vi "Xsens DT Parser (SubVI).vi"(5 "DT String In":string, 6 "DataType In":string) -> (0 "Channel Units":string[](array[string]), 1 "Channel DataTypes":string[](array[string]), 2 "Decoded Data Out":string[](array[string]), 3 "Channel Names":string[](array[string]))   [LabVIEW 2019]
doc: "This SubVI uses a state machine type structure to decode the XSens data measurement string based on the provided datatype. It outputs 4 fields that are contain the decoded data and metadata for writing to a TDMS file. \n\nAll data are output as strings. This is necessary to simplify the TDMS write function, since TDMS does not handle mixed data types (float, int, string, bool, etc) easily. \n\nCurrently, does not include decoders for all Xsens datatypes, however decoders can be easily added as need arises. \n\n2020 NREL"
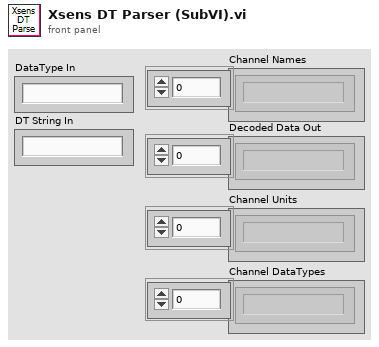
[diagram p1: front panel]
types:
  T1 = cluster{"Valid Time of Week":bool, "Valid Week Number":bool, "Valid UTC":bool}
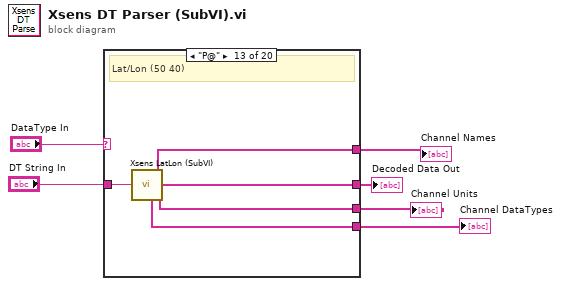
[diagram p0: block diagram]
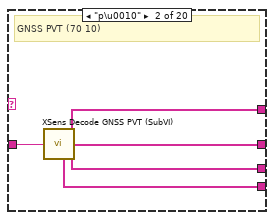
[diagram p3: hidden frame]
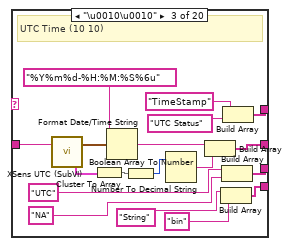
[diagram p4: hidden frame]
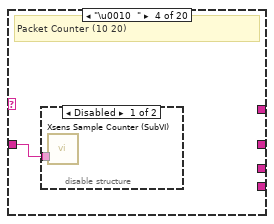
[diagram p5: hidden frame]
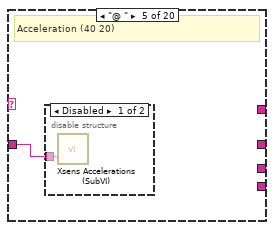
[diagram p7: hidden frame]
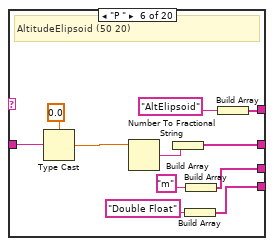
[diagram p9: hidden frame]
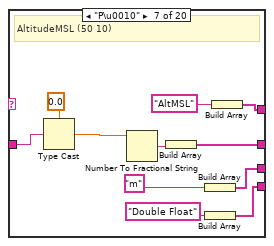
[diagram p10: hidden frame]
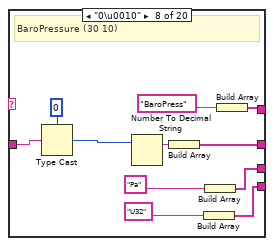
[diagram p11: hidden frame]
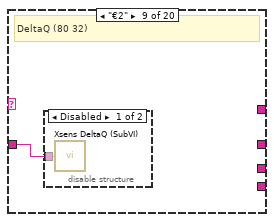
[diagram p12: hidden frame]
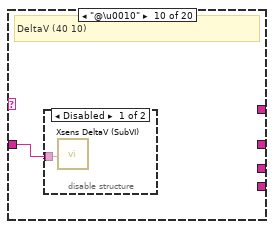
[diagram p14: hidden frame]
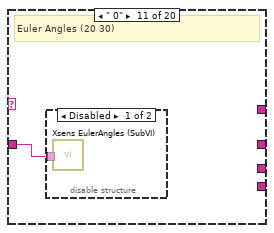
[diagram p16: hidden frame]
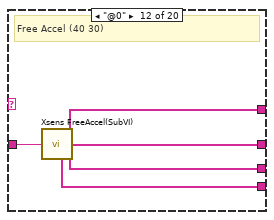
[diagram p18: hidden frame]
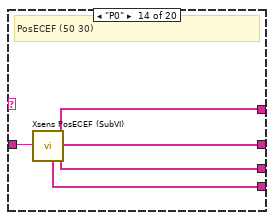
[diagram p19: hidden frame]
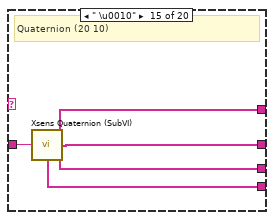
[diagram p20: hidden frame]
diagram:
  n1 = case shown="\"P@\"" "DataType In" {
    tunnel: "DT String In" -> [_ w11 w29 w30 w32 w43 w54 w65 w67 w69 w71 w77 w82 w87 w92 w97 w98 w100 w103 w110]
    tunnel: [_ w10 w26 _ _ w40 w51 w62 _ _ _ w76 w81 w83 w91 w96 _ _ _ w109] -> w3
    tunnel: [_ w9 w19 _ _ w38 w47 w58 _ _ _ w75 w80 w86 w90 w95 _ _ _ w108] -> w4
    tunnel: [_ w7 w15 _ _ w34 w45 w56 _ _ _ w73 w79 w84 w88 w93 _ _ _ w106] -> w1
    tunnel: [_ w8 w17 _ _ w35 w46 w57 _ _ _ w74 w78 w85 w89 w94 _ _ _ w107] -> w2
    frame "False", Default {
    }
    frame "p\u0010" {
      # "GNSS PVT (70 10)"
      n2 = call "XSens Decode GNSS PVT (SubVI).vi"("DATA In (Hex )"=w11) -> ("Channel Units"=w8:string[], "Channel DataTypes"=w7:string[], "GPS PVT out"=w10:string[], "Channel Names"=w9:string[])  [unwired: 1 out]
    }
    frame "\u0010\u0010" {
      # "UTC Time (10 10)"
      n3 = call "XSens UTC (SubVI).vi"("DATA In (Hex)"=w29) -> ("UTC Time"=w28:timestamp, "UTC Time Status"=w24:T1)
      n4 = Cluster To Array(cluster=w24) -> (array=w23:bool[])
      n5 = Format Date/Time String(time format string (%c)="%Y%m%d-%H:%M:%S%6u", seconds (now)=w28) -> (date/time string=w27:string)  [unwired: 1 in]
      n6 = Boolean Array To Number(Boolean array=w23) -> (number=w21:u32)
      n7 = Number To Decimal String(number=w21) -> (decimal integer string=w22:string)  [unwired: 1 in]
      n8 = Build Array(w27, w22) -> (w26:string[])
      n9 = Build Array("String", "bin") -> (w15:string[])
      n10 = Build Array("UTC", "NA") -> (w17:string[])
      n11 = Build Array("TimeStamp", "UTC Status") -> (w19:string[])
    }
    frame "\u0010  " {
      # "Packet Counter (10 20)"
      n12 = disable-structure shown="Disabled" {
        disable-tunnel: w30 -> [w31 _]
        frame Disabled {
          n13 = call "Xsens Sample Counter (SubVI).vi"("DATA In (Hex Display)"=w31) -> ()  [unwired: 1 out]
        }
        frame Enabled {
        }
      }
    }
    frame "@ " {
      # "Acceleration (40 20)"
      n14 = disable-structure shown="Disabled" {
        disable-tunnel: w32 -> [w33 _]
        frame Disabled {
          n15 = call "Xsens Accelerations (SubVI).vi"("DATA in (Hex)"=w33) -> ()  [unwired: 1 out]
        }
        frame Enabled {
        }
      }
    }
    frame "P " {
      # "AltitudeElipsoid (50 20)"
      n16 = Type Cast(type=sgl 0.0, x=w43) -> (*(type *) &x=w42:sgl)
      n17 = Number To Fractional String(number=w42) -> (F-format string=w41:string)  [unwired: 3 in]
      n18 = Build Array(w41) -> (w40:string[])
      n19 = Build Array("Double Float") -> (w34:string[])
      n20 = Build Array("m") -> (w35:string[])
      n21 = Build Array("AltElipsoid") -> (w38:string[])
    }
    frame "P\u0010" {
      # "AltitudeMSL (50 10)"
      n22 = Type Cast(type=sgl 0.0, x=w54) -> (*(type *) &x=w53:sgl)
      n23 = Number To Fractional String(number=w53) -> (F-format string=w52:string)  [unwired: 3 in]
      n24 = Build Array(w52) -> (w51:string[])
      n25 = Build Array("m") -> (w46:string[])
      n26 = Build Array("Double Float") -> (w45:string[])
      n27 = Build Array("AltMSL") -> (w47:string[])
    }
    frame "0\u0010" {
      # "BaroPressure (30 10)"
      n28 = Type Cast(type=u32 0, x=w65) -> (*(type *) &x=w64:u32)
      n29 = Number To Decimal String(number=w64) -> (decimal integer string=w63:string)  [unwired: 1 in]
      n30 = Build Array(w63) -> (w62:string[])
      n31 = Build Array("U32") -> (w56:string[])
      n32 = Build Array("Pa") -> (w57:string[])
      n33 = Build Array("BaroPress") -> (w58:string[])
    }
    frame "€2" {
      # "DeltaQ (80 32)"
      n34 = disable-structure shown="Disabled" {
        disable-tunnel: w67 -> [w68 _]
        frame Disabled {
          n35 = call "Xsens DeltaQ (SubVI).vi"("DATA in (Hex)"=w68) -> ()  [unwired: 1 out]
        }
        frame Enabled {
        }
      }
    }
    frame "@\u0010" {
      # "DeltaV (40 10)"
      n36 = disable-structure shown="Disabled" {
        disable-tunnel: w69 -> [w70 _]
        frame Disabled {
          n37 = call "Xsens DeltaV (SubVI).vi"("DATA in (Hex)"=w70) -> ()  [unwired: 1 out]
        }
        frame Enabled {
        }
      }
    }
    frame " 0" {
      # "Euler Angles (20 30)"
      n38 = disable-structure shown="Disabled" {
        disable-tunnel: w71 -> [w72 _]
        frame Disabled {
          n39 = call "Xsens EulerAngles (SubVI).vi"("DATA in (Hex)"=w72) -> ()  [unwired: 1 out]
        }
        frame Enabled {
        }
      }
    }
    frame "@0" {
      # "Free Accel (40 30)"
      n40 = call "Xsens FreeAccel(SubVI).vi"("DATA in (Hex)"=w77) -> ("Channel Units"=w74:string[], "Channel DataTypes"=w73:string[], "Decoded Data Out"=w76:string[], "Channel Names"=w75:string[])  [unwired: 1 in]
    }
    frame "P@" {
      # "Lat/Lon (50 40)"
      n41 = call "Xsens LatLon (SubVI).vi"("DATA in (Hex)"=w82) -> ("Channel Units"=w78:string[], "Channel DataTypes"=w79:string[], "Lat/Lon"=w81:string[], "Channel Names"=w80:string[])  [unwired: 1 in]
    }
    frame "P0" {
      # "PosECEF (50 30)"
      n42 = call "Xsens PosECEF (SubVI).vi"("DATA in (Hex)"=w87) -> ("Channel Units"=w85:string[], "Channel DataTypes"=w84:string[], "PosECEF"=w83:string[], "Channel Names"=w86:string[])  [unwired: 1 in]
    }
    frame " \u0010" {
      # "Quaternion (20 10)"
      n43 = call "Xsens Quaternion (SubVI).vi"("DATA in (Hex)"=w92) -> ("Channel Units"=w89:string[], "Channel DataTypes"=w88:string[], "Quaternion"=w91:string[], "Channel Names"=w90:string[])  [unwired: 1 in]
    }
    frame "€ " {
      # "Rate of Turn (80 20)"
      n44 = call "Xsens RateOfTurn (SubVI).vi"("DATA in (Hex)"=w97) -> ("Channel Units"=w94:string[], "Channel DataTypes"=w93:string[], "Rate of Turn"=w96:string[], "Channel Names"=w95:string[])  [unwired: 1 in]
    }
    frame "  " {
      # "Rotation Matrix"
      n45 = disable-structure shown="Disabled" {
        disable-tunnel: w98 -> [w99 _]
        frame Disabled {
          n46 = call "Xsens RotMatrix(SubVI).vi"("DATA in (Hex)"=w99) -> ()  [unwired: 1 out]
        }
        frame Enabled {
        }
      }
    }
    frame "\u0010`" {
      # "Sample Time Fine (10 60)"
      n47 = disable-structure shown="Disabled" {
        disable-tunnel: w100 -> [w101 _]
        frame Disabled {
          n48 = Type Cast(type=sgl 0.0, x=w101) -> ()  [unwired: 1 out]
        }
        frame Enabled {
        }
      }
    }
    frame "à\u0010" {
      # "Status Byte (E0 10)"
      n49 = disable-structure shown="Disabled" {
        disable-tunnel: w103 -> [w104 _]
        frame Disabled {
          n50 = Type Cast(type=u8 0, x=w104) -> ()  [unwired: 1 out]
        }
        frame Enabled {
        }
      }
    }
    frame "Ð\u0010" {
      # "Velocity (D0 10)"
      n51 = call "Xsens VelXYZ(SubVI).vi"("DATA in (Hex)"=w110) -> ("Channel Units"=w107:string[], "Channel DataTypes"=w106:string[], "Velocity"=w109:string[], "Channel Names"=w108:string[])  [unwired: 1 in]
    }
  }
  "Channel Names" <- w4
  "Decoded Data Out" <- w3
  "Channel Units" <- w2
  "Channel DataTypes" <- w1
